vi "Write Excel Files.vi"(5 "template file path":path=path "C:/Cascade/templates/Groundwater Profiling Log_empty_labview_template.xlsx", 6 "milliseconds \nto wait":u32=1000 min=800 max=2000, 7 "Header path":path=path "C:/Cascade/templates/Fields for Excel sheets.xlsx", 8 "error IO":errorcluster, 9 "Run  Loop":bool=TRUE, 10 "Output path to Directory":path=path "C:/Cascade/Data/Output Files/ara-1", 11 "Groundwater Header":T1={"Location"="Randolph", "Date Finished"="", "CTS"="", "sampler"="", "Kpro box Serial "="800", "Sonde Serial"="123456", "Drilling Contractor"="ara", "Ave Depth to Water"="", "Gas/Peri Pump"="Peri", "Atmospheric Pressure"="32", "KPRO N2 Pressure"="79", "Gas Drive N2 Pressure"="", "Profile ID"="ara-1", "Client"="ara"}) -> (0 "error out":errorcluster, 1 "Excel report file path":path=path "C:/Cascade/Data/Excel Reports/Groundwater Profiling Log_ara1.xlsx", 3 "NI_report out 2":refnum<class "NI_report.lvclass">)   [LabVIEW 2016]
uses:
  <vilib>/Utility/NIReport.llb/NI_report.lvclass
  sdi_12/Groundwater header.ctl
  Program Files/National Instruments/LabVIEW 2016/user.lib/_OpenG.lib/file/file.llb/Strip Path - Traditional__ogtk.vi
  Program Files/National Instruments/LabVIEW 2016/user.lib/_OpenG.lib/file/file.llb/Build Path - Traditional__ogtk.vi
  Program Files/National Instruments/LabVIEW 2016/user.lib/_OpenG.lib/file/file.llb/File Exists - Scalar__ogtk.vi
  <vilib>/Utility/file.llb/Write Delimited Spreadsheet (string).vi
  <vilib>/Utility/file.llb/Read Delimited Spreadsheet (string).vi
panel:
  in  "Serial Number/MISC":string
  in  "Groundwater header file":path
  out "header":bool
  in  "Read Groundwater Header File":bool
  in  "Clear Groundwater Header Values":bool
  out "Message":string
  out "Loop Indicator":i32
  in  "stop Data Entry Loop":bool
  out "Select Worksheet Index":i32
  in  "Sonde Calibration History File":path
  out "IK Reason array":string[][](array[string])
  out "Recording Reason Sonde array":string[][](array[string])
  in  "Temporary Data Files Directory":path=path "C:/Cascade/Data/Output Files"
  out "KPRO all rows":string[][](array[string])
  out "Sonde Data":string[][](array[string])
  out "Sonde Recording":string[][](array[string])
  out "IK":string[][](array[string])
  out "appended path":path=path "C:/Cascade/Data/Output Files/ara-1/ara-1"
  out "Down hole Pressure Transducer CSV data  path":path=path "C:/Cascade/Data/Output Files/ara-1/ara-1_DHT Data.csv"
  in  "Static IK path":path=path "C:/Cascade/Data/Output Files/ara-1/ara-1_Static Ik.csv"
  out "Output File Path":path=path "C:/Cascade/Data/Output Files/ara-1"
  out "KPRO SessionOutput File Path":path=path "C:/Cascade/Data/Output Files/ara-1/ara-1_KPROsession.csv"
  in  "Sonde Recording Error file":path=path "C:/Cascade/Data/Output Files/ara-1/ara-1_Sample failure.csv"
  in  "IK Recording Error file":path=path "C:/Cascade/Data/Output Files/ara-1/ara-1_IK failure.csv"
  in  "Sonde Output File Path":path=path "C:/Cascade/Data/Output Files/ara-1/ara-1_SondeData.csv"
  in  "KPRO Cumulative Output File Path":path=path "C:/Cascade/Data/Output Files/ara-1/ara-1_KPROcumulative.csv"
  out "Worksheet Names":string[](array[string])
  out "row max value":i32
  out "column max value":i32
  out "subarray":string[][](array[string])
  out "NI_report out":refnum<class "NI_report.lvclass">
  out "Number of Sample Sheets":i32
  out "Select Worksheet Index":i32
  out "Columns":i32[](array[numeric])
  out "Column of Volume":i32
  out "last occupied cell's name":string
  in  "Current  Sheet":string="Sample 1"
types:
  T1 = typedef "Groundwater header.ctl" = cluster{"Location":string, "Date Finished":string, "CTS":string, "sampler":string, "Kpro box Serial ":string, "Sonde Serial":string, "Drilling Contractor":string, "Ave Depth to Water":string, "Gas/Peri Pump":string, "Atmospheric Pressure":string, "KPRO N2 Pressure":string, "Gas Drive N2 Pressure":string, "Profile ID":string, "Client":string}
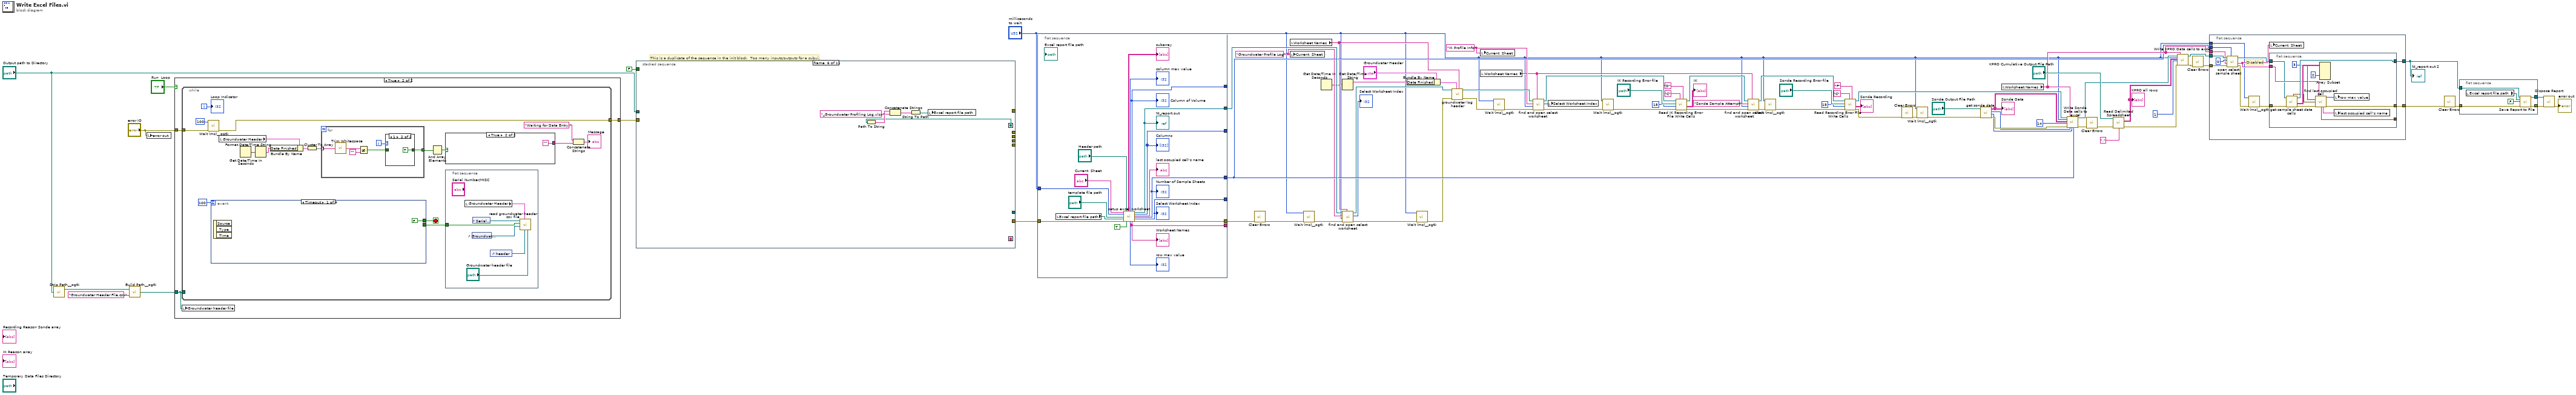
[diagram p0: block diagram]
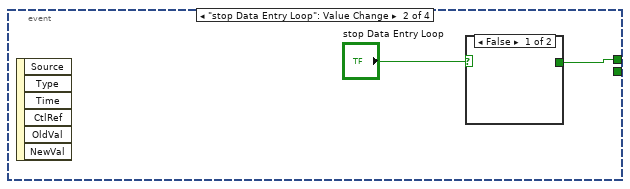
[diagram p3: hidden frame]
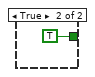
[diagram p4: hidden frame]
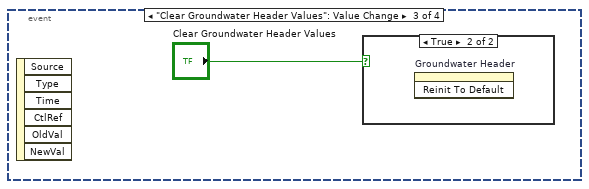
[diagram p5: hidden frame]
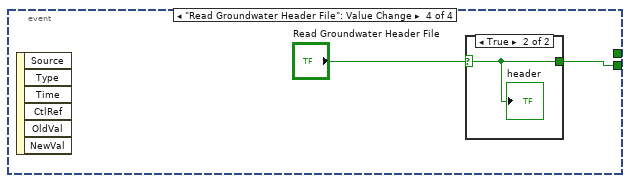
[diagram p7: hidden frame]
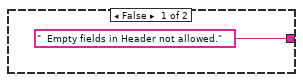
[diagram p9: hidden frame]
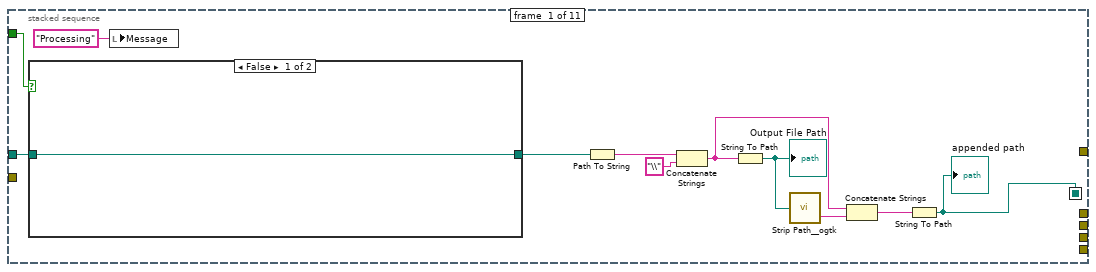
[diagram p11: hidden frame]
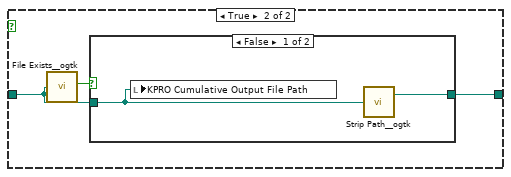
[diagram p12: hidden frame]
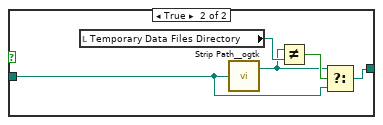
[diagram p13: hidden frame]
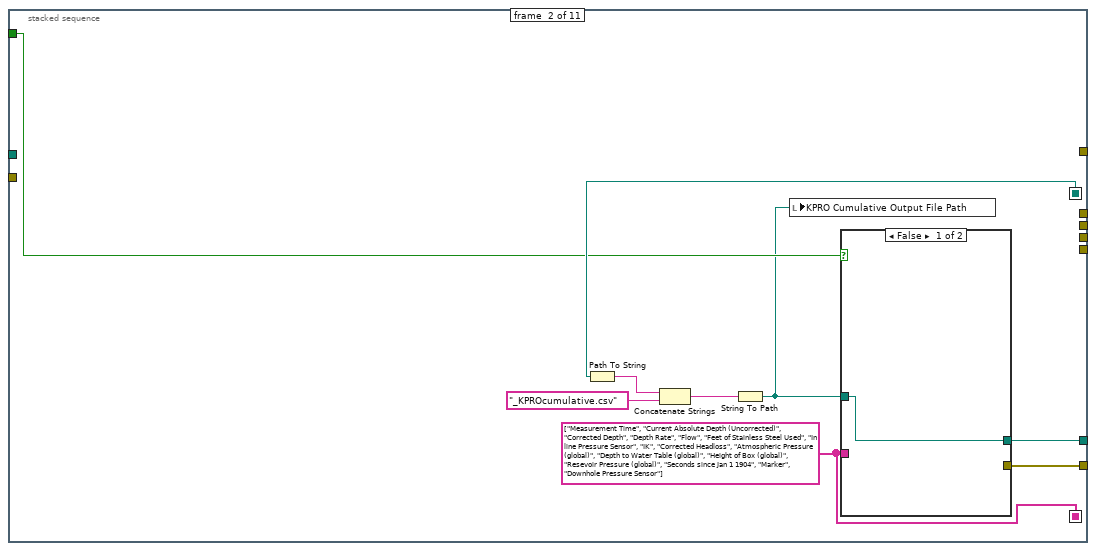
[diagram p14: hidden frame]
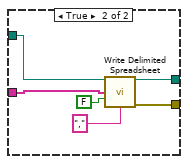
[diagram p15: hidden frame]
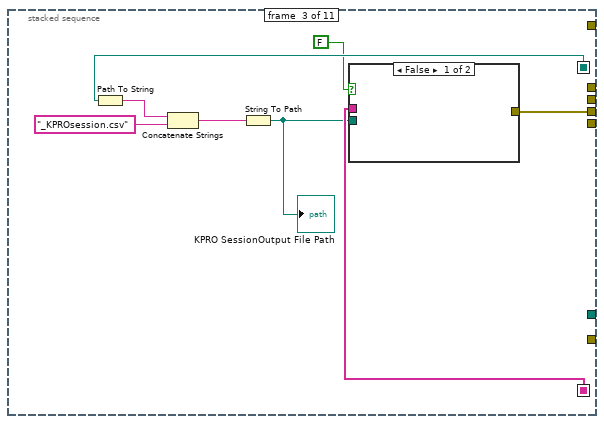
[diagram p16: hidden frame]
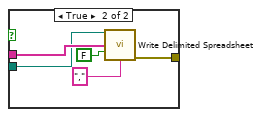
[diagram p17: hidden frame]
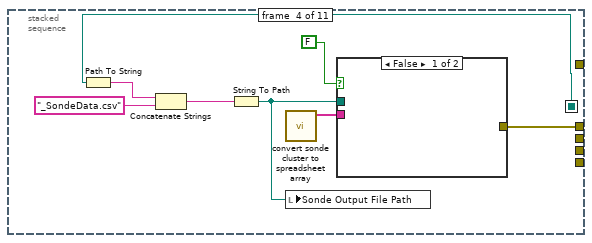
[diagram p18: hidden frame]
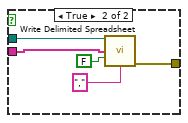
[diagram p19: hidden frame]
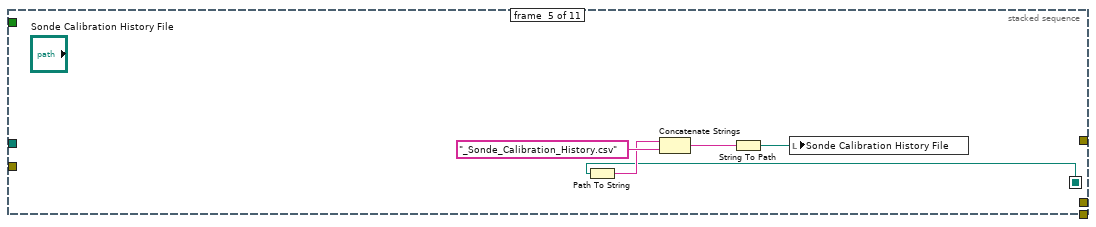
[diagram p20: hidden frame]
diagram:
  w39 = "Groundwater Profile Log" ("Worksheet Name in")
  w50 = "IK Profile Info" ("Worksheet Name in")
  # "This is a duplicate of the sequence in the init block.  Too many inputs/outputs for a subvi."
  n1 = call-poly "Strip Path__ogtk.vi"("path"="Output path to Directory") -> ("stripped path"=w1:path)  [unwired: 1 out]
  n2 = call-poly "Build Path__ogtk.vi"("name or relative path"="Groundwater Header File.csv", "base path"=w1) -> ("appended path"=w2:path)
  n3 = local write "error out"("error IO") -> ()
  n4 = case shown="True" "Run  Loop" {
    tunnel: "error IO" -> [w79 w82]
    tunnel: [w79 w81] -> w10
    tunnel: w2 -> [_ w80]
    frame False {
    }
    frame True {
      n5 = while {
        tunnel: w82 -> [w99]
        tunnel: [w89] -> w81
        tunnel: w80 -> [_]
        i -> [w97]
        stop <- w84 stop-if-true
        n6 = call "Wait (ms)__ogtk.vi"("error in (no error)"=w99, "milliseconds to wait"=u32 100) -> ("error out"=w89:errorcluster)  [unwired: 8 in, 1 out]
        n7 = event shown="[0] Timeout" {
          selector: _ -> [_ _ _ _]
          dyn-events: _ -> [_ _ _ _]
          timeout: 100 -> [_ _ _ _]
          tunnel: [FALSE w101 _ _] -> w84
          tunnel: [_ _ _ w105] -> w83
          event Timeout {
            n8 = event-data() -> ()  [unwired: 1 in, 3 out]
          }
          event "stop Data Entry Loop": Value Change {
            n9 = event-data() -> ()  [unwired: 1 in, 6 out]
            n10 = case shown="False" "stop Data Entry Loop" {
              tunnel: [_ TRUE] -> w101
              frame False {
              }
              frame True {
              }
            }
          }
          event "Clear Groundwater Header Values": Value Change {
            n11 = event-data() -> ()  [unwired: 1 in, 6 out]
            n12 = case shown="True" "Clear Groundwater Header Values" {
              frame False {
              }
              frame True {
                n13 = invoke on="Groundwater Header" class="Clust (strict)" method="Reinit To Default"() -> ()  [unwired: 3 in, 3 out]
              }
            }
          }
          event "Read Groundwater Header File": Value Change {
            n14 = event-data() -> ()  [unwired: 1 in, 6 out]
            n15 = case shown="True" "Read Groundwater Header File" {
              selector: "Read Groundwater Header File" -> [_ w107]
              tunnel: [_ w107] -> w105
              frame False {
              }
              frame True {
                "header" <- w107
              }
            }
          }
        }
        n16 = local read "Groundwater Header"() -> (w90:T1)
        n17 = Get Date/Time In Seconds() -> (seconds since 1Jan1904=w91:timestamp)
        n18 = Format Date/Time String(seconds (now)=w91) -> (date/time string=w92:string)  [unwired: 2 in]
        n19 = Bundle By Name(cluster=w90, "Date Finished"=w92) -> (w93:T1)
        n20 = Cluster To Array(cluster=w93) -> (array=w95:string[])
        n21 = for {
          tunnel: w95 -> [w115] mode=indexing
          tunnel: [w110] -> w94 mode=indexing
          i -> [w112]
          n22 = call <vilib>:"Trim Whitespace.vi"("string"=w115) -> ("trimmed string"=w114:string)  [unwired: 1 in]
          n23 = Not Equal?(x=w114, y="") -> (x != y?=w111:bool)
          n24 = case shown="1" w112 {
            tunnel: w111 -> [w116 _]
            tunnel: [w116 TRUE] -> w110
            frame 0, Default {
            }
            frame 1 {
            }
          }
        }
        n25 = And Array Elements(Boolean array=w94) -> (logical AND=w87:bool)
        n26 = case shown="True" w87 {
          tunnel: ["  Empty fields in Header not allowed." ""] -> w86
          frame False {
          }
          frame True {
          }
        }
        n27 = flat-sequence {
          tunnel: w83 -> [w118]
          frame #0 {
            n28 = local read "Groundwater Header"() -> (w123:T1)
            n29 = control-ref of="Groundwater Header"() -> (w120:refnum<vi>)
            n30 = control-ref of="Serial Number/MISC"() -> (w119:refnum<vi>)
            n31 = control-ref of="header"() -> (w122:refnum<vi>)
            n32 = call "read groundwater header csv file.vi"("Groundwater header file"="Groundwater header file", "header indicator reference 3"=w122, "Groundwater Header"=w123, "Groundwater Cluster reference in"=w120, "Read Groundwater Header File"=w118, "Sonde Serial Number String in"=w119) -> ()  [unwired: 6 in]
          }
        }
        n33 = Concatenate Strings("Waiting for Data Entry." ("Message"), w86) -> (→"Message":string)
        "Loop Indicator" <- w97
      }
      n34 = local write "Groundwater header file"(w80) -> ()
    }
  }
  n35 = stacked-sequence {
    seq-local: [_ w149 _ _ _ _ _ _ _ _ _] -> [_ _ w164 _ _ _ _ _ _ _ _]
    seq-local: [w125 _ _ _ _ _ _ _ _ _ _] -> [_ w150 w165 w177 w188 w193 w204 w220 w231 w235 _]
    tunnel: [_ w147 _ _ _ _ _ _ _ _ _] -> w29
    tunnel: [_ _ w169 _ _ _ _ _ _ _ _] -> _
    tunnel: [_ _ _ w178 _ _ _ _ _ _ _] -> _
    tunnel: [_ _ _ _ _ _ w205 _ _ _ _] -> _
    tunnel: [_ _ _ _ _ _ _ w221 _ _ _] -> _
    tunnel: [_ _ _ _ _ _ _ _ _ _ w242] -> _
    tunnel: [_ w151 _ _ _ _ _ _ _ _ _] -> _
    tunnel: "Output path to Directory" -> [w128 _ _ _ _ _ _ _ _ _ _]
    tunnel: FALSE ("exists") -> [w129 w148 _ _ _ _ _ _ _ _ _]
    tunnel: w10 -> [_ _ _ _ _ _ _ _ _ _ _]
    frame #0 {
      n36 = case shown="False" w129 {
        tunnel: w128 -> [w135 w137]
        tunnel: [w135 w136] -> w127
        frame False {
        }
        frame True {
          n37 = call-poly "File Exists__ogtk.vi"("file path"=w137) -> ("is directory"=w138:bool)  [unwired: 6 in, 1 out]
          n38 = case shown="False" w138 {
            tunnel: w137 -> [w139 w141]
            tunnel: [w140 w142] -> w136
            frame False {
              n39 = local write "KPRO Cumulative Output File Path"(w139) -> ()
              n40 = call-poly "Strip Path__ogtk.vi"("path"=w139) -> ("stripped path"=w140:path)  [unwired: 1 out]
            }
            frame True {
              n41 = local read "Temporary Data Files Directory"() -> (w145:path)
              n42 = call-poly "Strip Path__ogtk.vi"("path"=w141) -> ("stripped path"=w143:path)  [unwired: 1 out]
              n43 = Not Equal?(x=w143, y=w145) -> (x != y?=w144:bool)
              n44 = Select(t=w143, s=w144, f=w141) -> (s? t:f=w142:path)
            }
          }
        }
      }
      n45 = local write "Message"("Processing" ("Message")) -> ()
      n46 = Path To String(path=w127) -> (string=w132:string)
      n47 = Concatenate Strings(w132, "\\" ("string")) -> (w133:string)
      n48 = String To Path(string=w133) -> (path=w126:path)
      "Output File Path" <- w126
      n49 = call-poly "Strip Path__ogtk.vi"("path"=w126) -> ("name"=w130:string)  [unwired: 1 out]
      n50 = Concatenate Strings(w133, w130) -> (w131:string)
      n51 = String To Path(string=w131) -> (path=w125:path)
      "appended path" <- w125
    }
    frame #1 {
      w149 = string[] ["Measurement Time", "Current Absolute Depth (Uncorrected)", "Corrected Depth", "Depth Rate", "Flow", "Feet of Stainless Steel Used", "In line Pressure Sensor", "IK", "Corrected Headloss", "Atmospheric Pressure (global)", "Depth to Water Table (global)", "Height of Box (global)", "Resevoir Pressure (global)", "Seconds since Jan 1 1904", "Marker", "Downhole Pressure Sensor"] ("Array")
      n52 = Path To String(path=w150) -> (string=w152:string)
      n53 = Concatenate Strings(w152, "_KPROcumulative.csv") -> (w154:string)
      n54 = String To Path(string=w154) -> (path=w146:path)
      n55 = local write "KPRO Cumulative Output File Path"(w146) -> ()
      n56 = case shown="False" w148 {
        tunnel: [_ w159] -> w147
        tunnel: w146 -> [w155 w158]
        tunnel: [w155 w157] -> w151
        tunnel: w149 -> [_ w156]
        frame False {
        }
        frame True {
          n57 = call-poly <vilib>:"Write Delimited Spreadsheet.vi"("file path (dialog if empty)"=w158, "1D data"=w156, "append to file? (new file:F)"=FALSE, "delimiter (\\t)"="," ("delimiter (\\t)")) -> ("new file path (Not A Path if cancelled)"=w157:path, "error out"=w159:errorcluster)  [unwired: 10 in]
        }
      }
    }
    frame #2 {
      n58 = Path To String(path=w165) -> (string=w167:string)
      n59 = Concatenate Strings(w167, "_KPROsession.csv") -> (w168:string)
      n60 = String To Path(string=w168) -> (path=w163:path)
      "KPRO SessionOutput File Path" <- w163
      n61 = case shown="False" FALSE {
        tunnel: [_ w172] -> w169
        tunnel: w164 -> [_ w171]
        tunnel: w163 -> [_ w170]
        frame False {
        }
        frame True {
          n62 = call-poly <vilib>:"Write Delimited Spreadsheet.vi"("file path (dialog if empty)"=w170, "1D data"=w171, "append to file? (new file:F)"=FALSE, "delimiter (\\t)"="," ("delimiter (\\t)")) -> ("error out"=w172:errorcluster)  [unwired: 10 in, 1 out]
        }
      }
    }
    frame #3 {
      n63 = Path To String(path=w177) -> (string=w180:string)
      n64 = Concatenate Strings(w180, "_SondeData.csv" ("string")) -> (w181:string)
      n65 = String To Path(string=w181) -> (path=w176:path)
      n66 = call "convert sonde cluster to spreadsheet array.vi"() -> ("sonde labels"=w179:string[])  [unwired: 8 in, 3 out]
      n67 = local write "Sonde Output File Path"(w176) -> ()
      n68 = case shown="False" FALSE {
        tunnel: w179 -> [_ w187]
        tunnel: [_ w184] -> w178
        tunnel: w176 -> [_ w183]
        frame False {
        }
        frame True {
          n69 = call-poly <vilib>:"Write Delimited Spreadsheet.vi"("file path (dialog if empty)"=w183, "1D data"=w187, "append to file? (new file:F)"=FALSE, "delimiter (\\t)"="," ("delimiter (\\t)")) -> ("error out"=w184:errorcluster)  [unwired: 10 in, 1 out]
        }
      }
    }
    frame #4 {
      n70 = Path To String(path=w188) -> (string=w190:string)
      n71 = Concatenate Strings(w190, "_Sonde_Calibration_History.csv" ("string")) -> (w191:string)
      n72 = String To Path(string=w191) -> (path=w189:path)
      n73 = local write "Sonde Calibration History File"(w189) -> ()
    }
    frame #5 {
      n74 = Path To String(path=w193) -> (string=w195:string)
      n75 = Concatenate Strings(w195, "_Groundwater Profiling Log.xlsx" ("string")) -> (w196:string)
      n76 = String To Path(string=w196) -> (path=w194:path)
      n77 = local write "Excel report file path"(w194) -> ()
    }
    frame #6 {
      w201 = string[] ["Time", "Head Pressure", "Depth", "Select Entry Value", "Select Entry String"]
      n78 = local read "Recording Reason Sonde array"() -> (w202:string[][])
      n79 = Path To String(path=w204) -> (string=w206:string)
      n80 = Concatenate Strings(w206, "_Sample failure.csv" ("new ending (none)")) -> (w207:string)
      n81 = Insert Into Array(array=w202, index (row)=0, new element=w201) -> (w203:string[][])  [unwired: 1 in]
      n82 = String To Path(string=w207) -> (path=w199:path)
      n83 = local write "Recording Reason Sonde array"(w203) -> ()
      n84 = local write "Sonde Recording Error file"(w199) -> ()
      n85 = case shown="False" FALSE {
        tunnel: [_ w211] -> w205
        tunnel: w201 -> [_ w210]
        tunnel: w199 -> [_ w209]
        frame False {
        }
        frame True {
          n86 = call-poly <vilib>:"Write Delimited Spreadsheet.vi"("file path (dialog if empty)"=w209, "1D data"=w210, "append to file? (new file:F)"=FALSE, "delimiter (\\t)"="," ("delimiter (\\t)")) -> ("error out"=w211:errorcluster)  [unwired: 10 in, 1 out]
        }
      }
    }
    frame #7 {
      w217 = string[] ["Time", "Head Pressure", "Depth", "Select Entry Value", "Select Entry String", "Flow", "Feet of Stainless Steel Used", "Corrected Pressure", "Ik"]
      n87 = Path To String(path=w220) -> (string=w222:string)
      n88 = Concatenate Strings(w222, "_IK failure.csv" ("new ending (none)")) -> (w223:string)
      n89 = local read "IK Reason array"() -> (w218:string[][])
      n90 = String To Path(string=w223) -> (path=w215:path)
      n91 = local write "IK Recording Error file"(w215) -> ()
      n92 = case shown="False" FALSE {
        tunnel: [_ w227] -> w221
        tunnel: w217 -> [_ w226]
        tunnel: w215 -> [_ w225]
        frame False {
        }
        frame True {
          n93 = call-poly <vilib>:"Write Delimited Spreadsheet.vi"("file path (dialog if empty)"=w225, "1D data"=w226, "append to file? (new file:F)"=FALSE, "delimiter (\\t)"="," ("delimiter (\\t)")) -> ("error out"=w227:errorcluster)  [unwired: 10 in, 1 out]
        }
      }
      n94 = Insert Into Array(array=w218, index (row)=0, new element=w217) -> (w219:string[][])  [unwired: 1 in]
      n95 = local write "IK Reason array"(w219) -> ()
    }
    frame #8 {
      n96 = local write "appended path"(w231) -> ()
      n97 = Path To String(path=w231) -> (string=w232:string)
      n98 = Concatenate Strings(w232, "_DHT Data.csv" ("new ending (none)")) -> (w233:string)
      n99 = String To Path(string=w233) -> (path=→"Down hole Pressure Transducer CSV data  path":path)
    }
    frame #9 {
      n100 = Path To String(path=w235) -> (string=w236:string)
      n101 = Concatenate Strings(w236, "_Static Ik.csv" ("string")) -> (w238:string)
      n102 = String To Path(string=w238) -> (path=w237:path)
      n103 = local write "Static IK path"(w237) -> ()
    }
    frame #10 {
      n104 = Build Array("Profile ID   " ("string"), "Depth    " ("string"), "Flow " ("string"), "Ik    " ("string")) -> (w243:string[])
      n105 = case shown="True" FALSE {
        tunnel: w243 -> [_ w251]
        tunnel: [_ w249] -> w242
        tunnel: "Static IK path" -> [_ w248]
        frame False {
        }
        frame True {
          n106 = call-poly <vilib>:"Write Delimited Spreadsheet.vi"("file path (dialog if empty)"=w248, "1D data"=w251, "append to file? (new file:F)"=FALSE, "delimiter (\\t)"="," ("delimiter (\\t)")) -> ("error out"=w249:errorcluster)  [unwired: 10 in, 1 out]
        }
      }
    }
  }
  n107 = flat-sequence {
    tunnel: [w269] -> w59
    tunnel: [w268] -> _
    tunnel: [w259] -> _
    tunnel: [w267] -> _
    tunnel: [w266] -> w78
    tunnel: [w265] -> w77
    tunnel: [w263] -> _
    tunnel: w29 -> [w257]
    tunnel: "milliseconds \nto wait" -> [w253]
    frame #0 {
      n108 = local read "Excel report file path"() -> (w254:path)
      n109 = call "setup excel worksheet.vi"("Current Sample Sheet"="Current  Sheet", "milliseconds to wait"=w253, "template file path"="template file path", "Excel report file path"=w254, "error in (no error)"=w257, "Header path"="Header path", "Open Excel Files"=TRUE) -> ("subarray"=→"subarray":string[][], "column max value"=→"column max value":i32, "row max value"=→"row max value":i32, "Column of Volume"=w263:i32, "Worksheet Names"=w259:string[], "NI_report out"=w266:refnum<class "NI_report.lvclass">, "Columns"=w268:i32[], "start of last occupied row"=→"last occupied cell's name":string, "Number of Sample Sheets"=w269:i32, "Select Worksheet Index"=w267:i32, "error out"=w265:errorcluster)  [unwired: 2 in]
      "Worksheet Names" <- w259
      "NI_report out" <- w266
      "Number of Sample Sheets" <- w269
      "Select Worksheet Index" <- w267
      "Columns" <- w268
      "Column of Volume" <- w263
    }
  }
  n110 = call <vilib>:"Clear Errors.vi"("error in (no error)"=w77) -> ("error out"=w31:errorcluster)  [unwired: 5 in, 1 out]
  n111 = local read "Worksheet Names"() -> (w38:string[])
  n112 = local write "Current  Sheet"(w39) -> ()
  n113 = call "Wait (ms)__ogtk.vi"("error in (no error)"=w31, "milliseconds to wait"="milliseconds \nto wait") -> ("error out"=w18:errorcluster)  [unwired: 8 in, 1 out]
  n114 = Get Date/Time In Seconds() -> (seconds since 1Jan1904=w35:timestamp)
  n115 = Get Date/Time String(seconds (now)=w35) -> (date string=w33:string)  [unwired: 2 in, 1 out]
  n116 = call "find and open select worksheet.vi"("Worksheet Names"=w38, "error in (no error)"=w18, "milliseconds to wait"="milliseconds \nto wait", "Worksheet Name in"=w39, "NI_report in"=w78) -> ("error out"=w37:errorcluster, "Select Worksheet Index"=→"Select Worksheet Index":i32, "NI_report out"=w36:refnum<class "NI_report.lvclass">)  [unwired: 4 in]
  n117 = Bundle By Name(cluster="Groundwater Header", "Date Finished"=w33) -> (w34:T1)
  n118 = call "Wait (ms)__ogtk.vi"("error in (no error)"=w37, "milliseconds to wait"="milliseconds \nto wait") -> ("error out"=w17:errorcluster)  [unwired: 8 in, 1 out]
  n119 = call "groundwater log header.vi"("Worksheet Names"=w38, "Groundwater Header"=w34, "error in (no error)"=w17, "NI_report in"=w36) -> ("error out"=w8:errorcluster, "NI_report out"=w74:refnum<class "NI_report.lvclass">)  [unwired: 6 in]
  n120 = local write "Current  Sheet"(w50) -> ()
  n121 = local read "Worksheet Names"() -> (w28:string[])
  n122 = call "Wait (ms)__ogtk.vi"("error in (no error)"=w8, "milliseconds to wait"="milliseconds \nto wait") -> ("error out"=w7:errorcluster)  [unwired: 8 in, 1 out]
  n123 = call "find and open select worksheet.vi"("Worksheet Names"=w28, "error in (no error)"=w7, "milliseconds to wait"="milliseconds \nto wait", "Worksheet Name in"=w50, "NI_report in"=w74) -> ("error out"=w16:errorcluster, "Select Worksheet Index"=w21:i32, "NI_report out"=w46:refnum<class "NI_report.lvclass">)  [unwired: 4 in]
  n124 = local write "Select Worksheet Index"(w21) -> ()
  n125 = call "Wait (ms)__ogtk.vi"("error in (no error)"=w16, "milliseconds to wait"="milliseconds \nto wait") -> ("error out"=w15:errorcluster)  [unwired: 8 in, 1 out]
  n126 = call "Read IK Recording Error File Write Cells.vi"("Reason Column Letter"="D", "Depth Column Letter"="C", "error in (no error)"=w15, "Row Offset In"=15, "IK Recording Data file"="IK Recording Error file", "NI_report in"=w46) -> ("error out"=w24:errorcluster, "all rows"=→"IK":string[][], "NI_report out"=w26:refnum<class "NI_report.lvclass">)  [unwired: 2 in, 1 out]
  n127 = call "find and open select worksheet.vi"("Worksheet Names"=w28, "error in (no error)"=w24, "milliseconds to wait"="milliseconds \nto wait", "Worksheet Name in"="Sonde Sample Attempt", "NI_report in"=w26) -> ("error out"=w14:errorcluster, "NI_report out"=w25:refnum<class "NI_report.lvclass">)  [unwired: 4 in, 1 out]
  n128 = call "Wait (ms)__ogtk.vi"("error in (no error)"=w14, "milliseconds to wait"="milliseconds \nto wait") -> ("error out"=w13:errorcluster)  [unwired: 8 in, 1 out]
  n129 = call "Read Recording Error File Write Cells.vi"("Reason Column Letter"="F", "Depth Column Letter"="C", "error in (no error)"=w13, "Row Offset In"=15, "Sonde Data file"="Sonde Recording Error file", "NI_report in"=w25) -> ("error out"=w67:errorcluster, "all rows"=→"Sonde Recording":string[][], "NI_report out"=w69:refnum<class "NI_report.lvclass">)  [unwired: 2 in, 1 out]
  n130 = call <vilib>:"Clear Errors.vi"("error in (no error)"=w67) -> ("error out"=w12:errorcluster)  [unwired: 5 in, 1 out]
  n131 = call "Wait (ms)__ogtk.vi"("error in (no error)"=w12, "milliseconds to wait"="milliseconds \nto wait") -> ("error out"=w11:errorcluster)  [unwired: 8 in, 1 out]
  n132 = call "get sonde data.vi"("error in (no error)"=w11, "Sonde Output File Path"="Sonde Output File Path") -> ("error out"=w66:errorcluster, "Sample Row \nBreak points"=w65:i32[], "Sample Array"=w58:i32[], "Sonde Data"=w68:string[][])  [unwired: 6 in]
  "Sonde Data" <- w68
  n133 = local read "Worksheet Names"() -> (w60:string[])
  n134 = call "Write Sonde Data cells to excel.vi"("NI_report in"=w69, "milliseconds to wait"="milliseconds \nto wait", "all rows"=w68, "Row Offset In"=14, "error in (no error)"=w66, "Worksheet Names"=w60, "Sample Array"=w58, "Sample Row \nBreak points"=w65, "Number of Sample Sheets"=w59) -> ("NI_report out"=w54:refnum<class "NI_report.lvclass">, "error out"=w63:errorcluster)  [unwired: 8 in, 1 out]
  n135 = call <vilib>:"Clear Errors.vi"("error in (no error)"=w63) -> ("error out"=w56:errorcluster)  [unwired: 5 in, 1 out]
  n136 = call-poly <vilib>:"Read Delimited Spreadsheet.vi"("file path (dialog if empty)"="KPRO Cumulative Output File Path", "error in (no error)"=w56, "delimiter (\\t)"="," ("delimiter (\\t)")) -> ("all rows"=w61:string[][], "error out"=w62:errorcluster)  [unwired: 7 in, 4 out]
  "KPRO all rows" <- w61
  n137 = call "Write KPRO Data cells to excel.vi"("NI_report in"=w54, "milliseconds to wait"="milliseconds \nto wait", "all rows"=w61, "Row Offset In"=1, "error in (no error)"=w62, "Worksheet Names"=w60) -> ("NI_report out"=w53:refnum<class "NI_report.lvclass">, "error out"=w57:errorcluster)  [unwired: 11 in, 1 out]
  n138 = call <vilib>:"Clear Errors.vi"("error in (no error)"=w57) -> ("error out"=w55:errorcluster)  [unwired: 5 in, 1 out]
  n139 = flat-sequence {
    tunnel: w55 -> [w282]
    tunnel: [w281] -> w76
    tunnel: w53 -> [w280]
    tunnel: [w279] -> w75
    tunnel: w59 -> [w275]
    tunnel: w60 -> [w273]
    tunnel: "milliseconds \nto wait" -> [w271]
    frame #0 {
      # "Disabled"
      n140 = call "open select sample sheet.vi"("Number of Sample Sheets"=w275, "error in (no error)"=w282, "Worksheet Names"=w273, "input 1"=0 ("Active Sample Sheet"), "NI_report in"=w280) -> ("error out"=w278:errorcluster, "Current Sample Sheet"=w274:string, "NI_report out"=w277:refnum<class "NI_report.lvclass">)  [unwired: 4 in]
      n141 = call "Wait (ms)__ogtk.vi"("error in (no error)"=w278, "milliseconds to wait"=w271) -> ("error out"=w272:errorcluster)  [unwired: 8 in, 1 out]
      n142 = local write "Current  Sheet"(w274) -> ()
      n143 = flat-sequence {
        tunnel: [w294] -> w279
        tunnel: [w293] -> _
        tunnel: w272 -> [w292]
        tunnel: [w285] -> w281
        tunnel: w274 -> [w284]
        tunnel: w277 -> [w283]
        frame #0 {
          n144 = call "get sample sheet data cells.vi"("error in (no error)"=w292, "NI_report in"=w283) -> ("error out"=w295:errorcluster, "data"=w290:string[][], "NI_report out"=w294:refnum<class "NI_report.lvclass">, "left edge output cluster"=w288:cluster{"row":i32, "column":i32})  [unwired: 5 in, 1 out]
          n145 = call "find last occupied cell.vi"("Active Sheet"=w284, "Header Rows to remove"=3, "sub array start"=w288, "error in (no error)"=w295) -> ("row max value"=w287:i32, 13:"start of last occupied row"=w293:cluster{"row":i32, "column":i32}, 14:"start of last occupied row"=w286:string, "error out"=w285:errorcluster)  [unwired: 5 in, 3 out]
          n146 = Array Subset(array=w290, index (col)=2 ("index")) -> ()  [unwired: 3 in, 1 out]
          n147 = local write "row max value"(w287) -> ()
          n148 = local write "last occupied cell's name"(w286) -> ()
        }
      }
    }
  }
  n149 = call <vilib>:"Clear Errors.vi"("error in (no error)"=w76) -> ("error out"=w32:errorcluster)  [unwired: 5 in, 1 out]
  n150 = flat-sequence {
    tunnel: [w301] -> w73
    tunnel: [w300] -> w72
    tunnel: w32 -> [w298]
    tunnel: w75 -> [w297]
    frame #0 {
      n151 = local read "Excel report file path"() -> (w296:path)
      n152 = call-dynamic "Save Report to File.vi"("report in"=w297, "report file path"=w296, "prompt to replace? (F)"=FALSE, "error in (no error)"=w298) -> ("report out"=w301:refnum<class "NI_report.lvclass">, "error out"=w300:errorcluster)  [unwired: 10 in]
    }
  }
  n153 = call-dynamic "Dispose Report.vi"("report in"=w73, "error in (no error)"=w72) -> ("error out"=→"error out":errorcluster)  [unwired: 13 in]
  "NI_report out 2" <- w75
